vi "Modbus Command Explainer.vi"() -> ()   [LabVIEW 2010]
panel:
  out "Array":u8[](array[numeric])
  out "Explanation":string
  in  "Modbus String":string
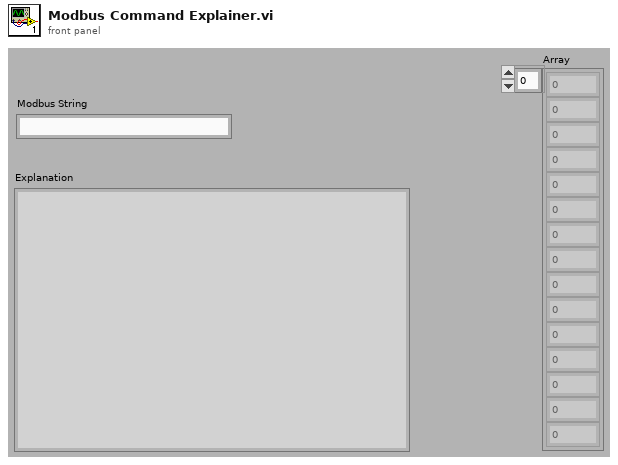
[diagram p1: front panel]
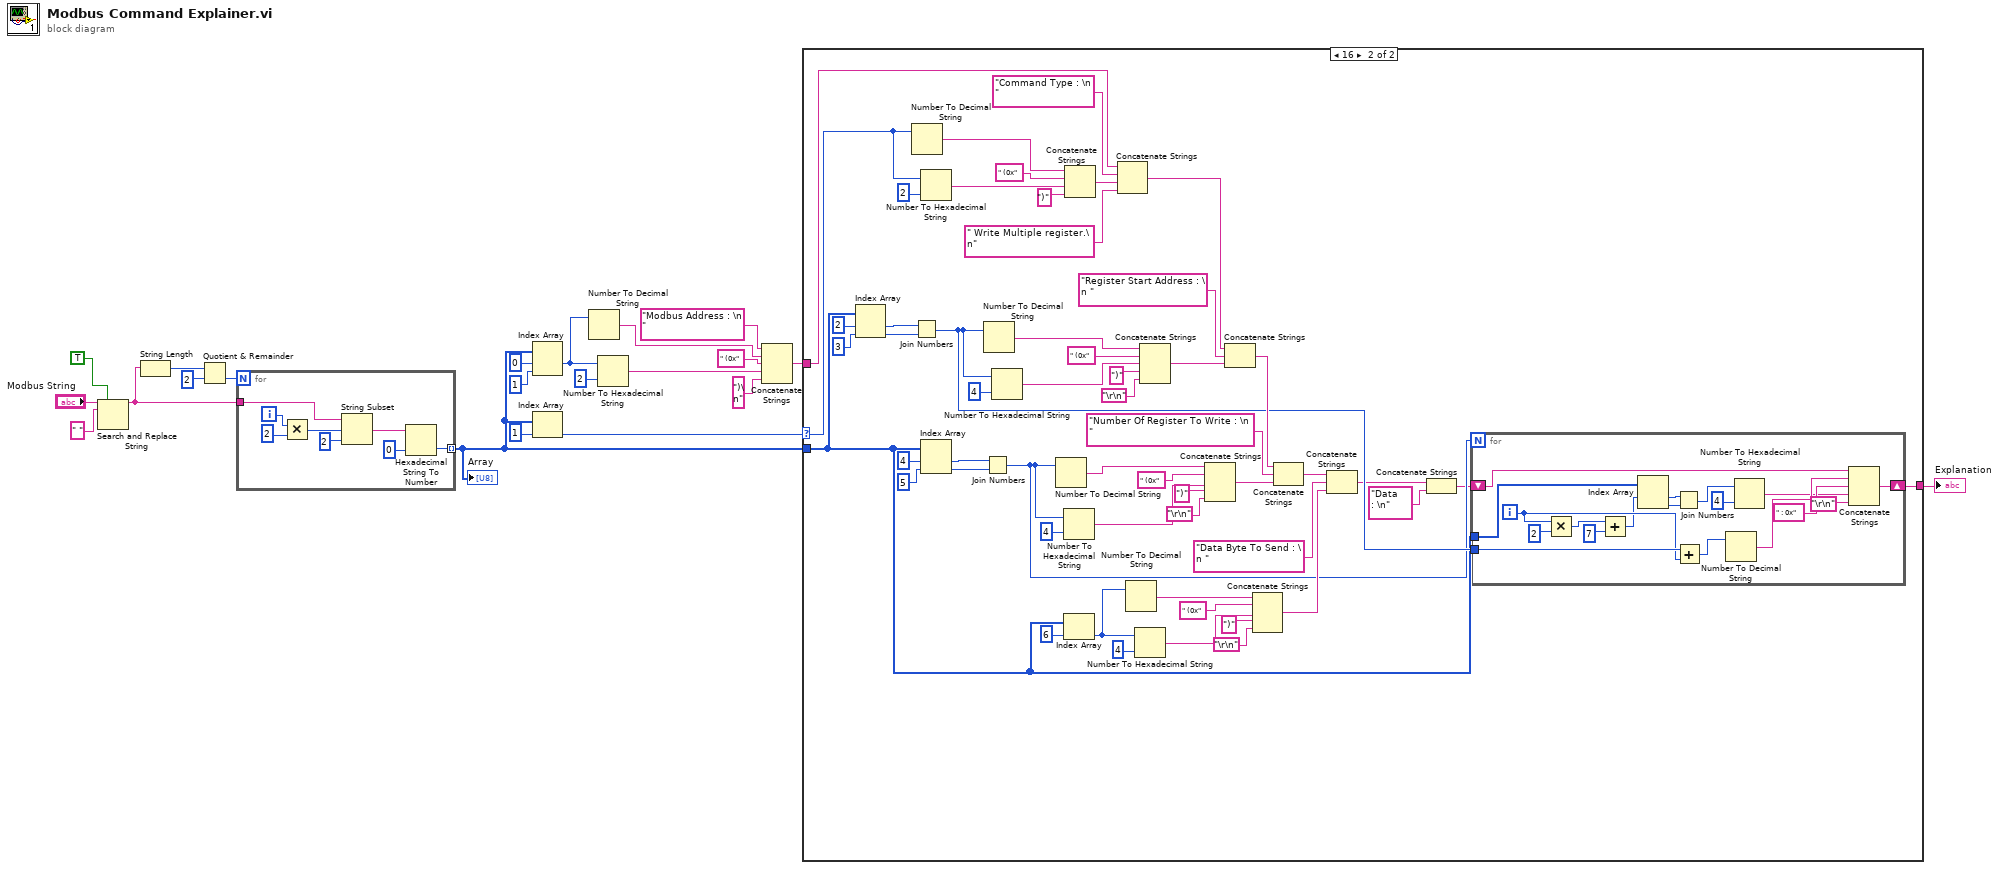
[diagram p0: block diagram]
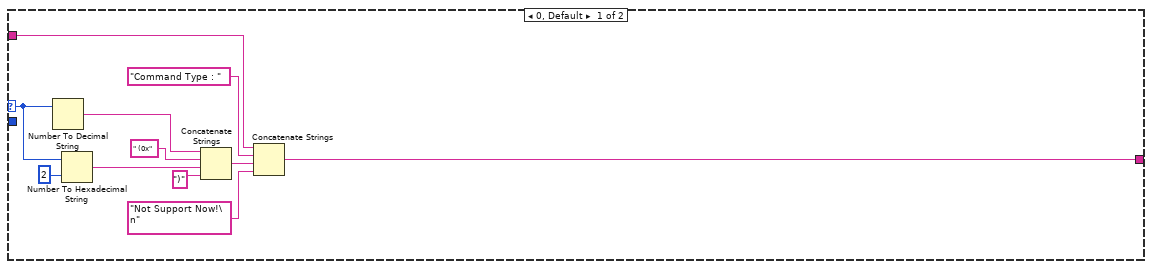
[diagram p2: hidden frame]
diagram:
  n1 = Search and Replace String(replace all?=TRUE ("replace all? (F)"), input string="Modbus String", search string=" ") -> (result string=w18:string)  [unwired: 5 in, 3 out]
  n2 = String Length(string=w18) -> (length=w17:i32)
  n3 = Quotient & Remainder(x=w17, y=2) -> (floor(x/y)=w16:i32)  [unwired: 1 out]
  n4 = for {
    N: w16 -> [_]
    tunnel: w18 -> [w25]
    tunnel: [w22] -> w1 mode=indexing
    i -> [w28]
    n5 = Multiply(x=w28, y=2 ("x")) -> (x*y=w27:i32)
    n6 = String Subset(string=w25, offset (0)=w27, length (rest)=2 ("length (rest)")) -> (substring=w23:string)
    n7 = Hexadecimal String To Number(string=w23, default (0uL)=u8 0 ("default (0 U32)")) -> (number=w22:u8)  [unwired: 1 in, 1 out]
  }
  "Array" <- w1
  n8 = Index Array(array=w1, index #1=0 ("index"), index #2=1 ("index")) -> (element #1=w11:u8)  [unwired: 1 out]
  n9 = Index Array(array=w1, index=1) -> (element=w2:u8)
  n10 = Number To Decimal String(number=w11) -> (decimal integer string=w13:string)  [unwired: 1 in]
  n11 = Number To Hexadecimal String(1:i16 2 ("width (-)"), 2:w11) -> (0:w9:string)
  n12 = Concatenate Strings("Modbus Address : \n " ("string"), w13, " (0x" ("string"), w9, ")\n" ("string")) -> (w5:string)
  n13 = case shown="16" w2 {
    selector: w2 -> [w32 w86]
    tunnel: w5 -> [w40 w94]
    tunnel: [w30 w41] -> w4
    tunnel: w1 -> [_ w45]
    frame 0, Default {
      n14 = Number To Decimal String(number=w32) -> (decimal integer string=w37:string)  [unwired: 1 in]
      n15 = Number To Hexadecimal String(1:i16 2 ("width (-)"), 2:w32) -> (0:w35:string)
      n16 = Concatenate Strings(w37, " (0x" ("string"), w35, ")" ("string")) -> (w31:string)
      n17 = Concatenate Strings(w40, "Command Type : " ("string"), w31, "Not Support Now!\n" ("string")) -> (w30:string)
    }
    frame 16 {
      n18 = Index Array(array=w45, index #1=2 ("index"), index #2=3 ("index")) -> (element #1=w82:u8, element #2=w81:u8)
      n19 = Number To Decimal String(number=w86) -> (decimal integer string=w91:string)  [unwired: 1 in]
      n20 = Join Numbers(hi=w82, lo=w81) -> ((hi.lo)=w47:u16)
      n21 = Number To Hexadecimal String(1:i16 2 ("width (-)"), 2:w86) -> (0:w89:string)
      n22 = Index Array(array=w45, index #1=4 ("index"), index #2=5 ("index")) -> (element #1=w62:u8, element #2=w63:u8)
      n23 = Join Numbers(hi=w62, lo=w63) -> ((hi.lo)=w46:u16)
      n24 = Number To Decimal String(number=w47) -> (decimal integer string=w75:string)  [unwired: 1 in]
      n25 = Number To Hexadecimal String(1:i16 4 ("width (-)"), 2:w47) -> (0:w77:string)
      n26 = Number To Decimal String(number=w46) -> (decimal integer string=w69:string)  [unwired: 1 in]
      n27 = Number To Hexadecimal String(1:i16 4 ("width (-)"), 2:w46) -> (0:w67:string)
      n28 = Index Array(array=w45, index=6) -> (element=w49:u8)
      n29 = Concatenate Strings(w91, " (0x" ("string"), w89, ")" ("string")) -> (w85:string)
      n30 = Concatenate Strings(w94, "Command Type : \n " ("string"), w85, " Write Multiple register.\n" ("string")) -> (w73:string)
      n31 = Number To Decimal String(number=w49) -> (decimal integer string=w52:string)  [unwired: 1 in]
      n32 = Number To Hexadecimal String(1:i16 4 ("width (-)"), 2:w49) -> (0:w54:string)
      n33 = Concatenate Strings(w75, " (0x" ("string"), w77, ")" ("string"), "\r\n") -> (w80:string)
      n34 = Concatenate Strings(w69, " (0x" ("string"), w67, ")" ("string"), "\r\n") -> (w64:string)
      n35 = Concatenate Strings(w73, "Register Start Address : \n " ("string"), w80) -> (w59:string)
      n36 = Concatenate Strings(w52, " (0x" ("string"), w54, ")" ("string"), "\r\n") -> (w57:string)
      n37 = Concatenate Strings(w59, "Number Of Register To Write : \n " ("string"), w64) -> (w48:string)
      n38 = Concatenate Strings(w48, "Data Byte To Send : \n " ("string"), w57) -> (w42:string)
      n39 = Concatenate Strings(w42, "Data  : \n" ("string")) -> (w43:string)
      n40 = for {
        N: w46 -> [_]
        tunnel: w47 -> [w112]
        tunnel: w45 -> [w111]
        shift-right: [w97] -> w41
        shift-left: w43 -> [w101]
        i -> [w110]
        n41 = Multiply(x=w110, y=2) -> (x*y=w96:i32)
        n42 = Add(x=w96, y=7) -> (x+y=w108:i32)
        n43 = Index Array(array=w111, index #1=w108) -> (element #1=w106:u8, element #2=w107:u8)  [unwired: 1 in]
        n44 = Join Numbers(hi=w106, lo=w107) -> ((hi.lo)=w103:u16)
        n45 = Add(x=w112, y=w110) -> (x+y=w105:i32)
        n46 = Number To Decimal String(number=w105) -> (decimal integer string=w102:string)  [unwired: 1 in]
        n47 = Number To Hexadecimal String(1:i16 4 ("width (-)"), 2:w103) -> (0:w99:string)
        n48 = Concatenate Strings(w101, w102, " : 0x" ("string"), w99, "\r\n") -> (w97:string)
      }
    }
  }
  "Explanation" <- w4
